vi "Parse Emission Current.vi"(1 "Numeric":i32) -> (0 "current (A)":dbl)   [LabVIEW 2019, in "PGC2D.lvlib"]
uses:
  PGC2D.lvlib
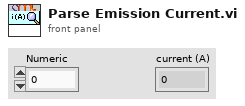
[diagram p1: front panel]
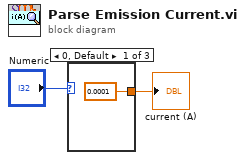
[diagram p0: block diagram]
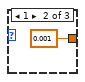
[diagram p2: hidden frame]
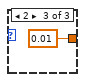
[diagram p3: hidden frame]
diagram:
  n1 = case shown="0, Default" "Numeric" {
    tunnel: [0.0001 ("x") 0.001 ("x") 0.01 ("x")] -> w1
    frame 0, Default {
    }
    frame 1 {
    }
    frame 2 {
    }
  }
  "current (A)" <- w1
